vi "Instantiate.vi"(11 "error in":errorcluster) -> (4 "function manager":refnum<class "function manager.lvclass">, 15 "error out":errorcluster)   [LabVIEW 2016, in "function manager.lvclass"]
uses:
  function manager.lvclass
  functionsbase/functionbase.lvclass
  function manager.lvclass/function manager.ctl
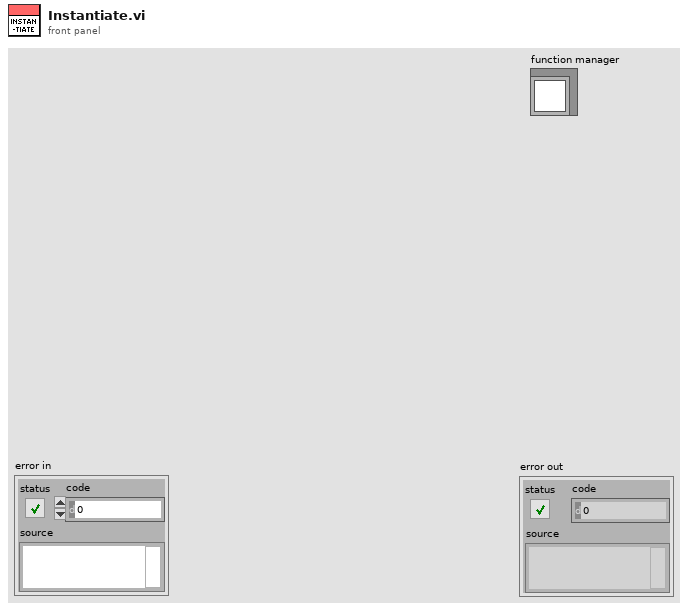
[diagram p1: front panel]
types:
  T1 = typedef "Scan Syntax Format.ctl" = cluster{"Syntax":string, "Variable#":i32, "Variables Name":string[]}
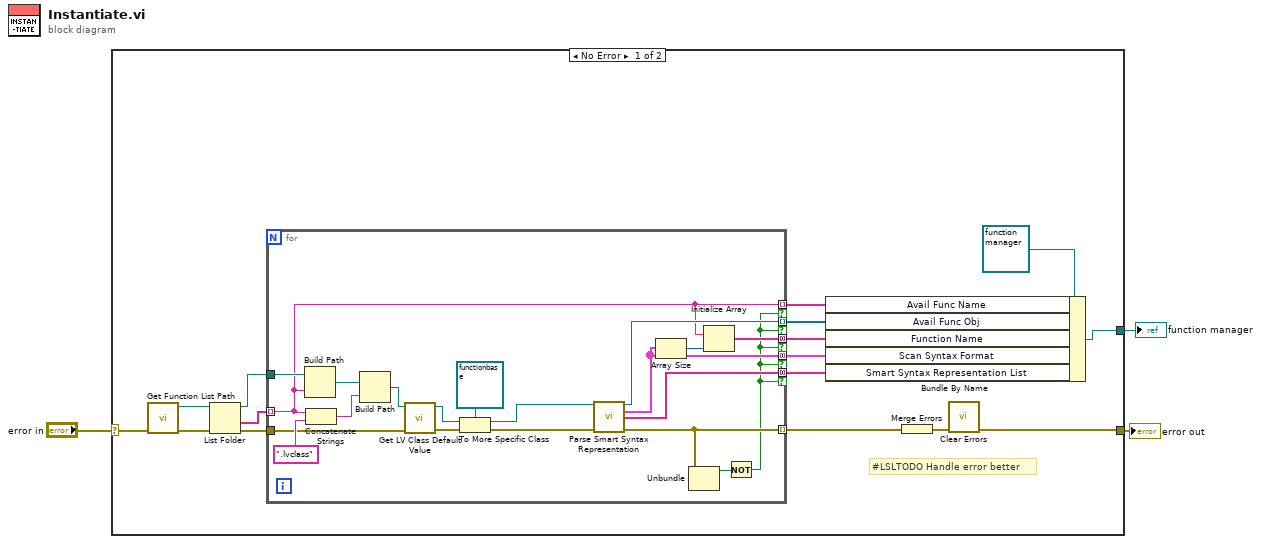
[diagram p0: block diagram]
diagram:
  n1 = case shown="No Error" "error in" {
    selector: "error in" -> [w19 w40]
    tunnel: [w11 w40] -> w2
    tunnel: [w7 _] -> w1
    frame No Error {
      # "#LSLTODO Handle error better"
      n2 = call "Get Function List Path.vi"("error in"=w19) -> ("error out"=w18:errorcluster, "Functions List Path"=w17:path)  [unwired: 9 in]
      n3 = List Folder(path=w17, error in=w18) -> (path out=w14:path, folder names=w15:string[], error out=w16:errorcluster)  [unwired: 2 in, 1 out]
      n4 = for {
        tunnel: w16 -> [w34]
        tunnel: w15 -> [w23] mode=indexing
        tunnel: w14 -> [w39]
        tunnel: [w28] -> w13 mode=indexing
        tunnel: [w26] -> w8 mode=indexing if=w20
        tunnel: [w23] -> w9 mode=indexing if=w20
        tunnel: [w25] -> w5 mode=concatenating if=w20
        tunnel: [w22] -> w6 mode=concatenating if=w20
        tunnel: [w21] -> w4 mode=concatenating if=w20
        n5 = Build Path(base path=w39, name or relative path=w23) -> (appended path=w38:path)
        n6 = Concatenate Strings(w23, ".lvclass" ("string")) -> (w36:string)
        n7 = Build Path(base path=w38, name or relative path=w36) -> (appended path=w35:path)
        n8 = call <vilib>:"Get LV Class Default Value.vi"("error in (no error)"=w34, "class path"=w35) -> ("error out"=w33:errorcluster, "object"=w32:refnum<class>)  [unwired: 8 in]
        n9 = To More Specific Class(target class=refnum<class "functionbase.lvclass"> refnum ("functionbase.lvclass"), reference=w32, error in=w33) -> (specific class reference=w27:refnum<class "functionbase.lvclass">, error out=w29:errorcluster)
        n10 = call-dynamic "Parse Smart Syntax Representation.vi"("functionbase in"=w27, "error in (no error)"=w29) -> ("functionbase out"=w26:refnum<class "functionbase.lvclass">, "Scan Syntax List"=w25:T1[], "Smart Syntax Representation List"=w21:string[], "error out"=w28:errorcluster)  [unwired: 10 in]
        n11 = Array Size(array=w25) -> (size(s)=w24:i32)
        n12 = Unbundle(w28) -> ("status"=w30:bool)  [unwired: 2 out]
        n13 = Initialize Array(w23, w24) -> (w22:string[])
        n14 = Not(x=w30) -> (.not. x?=w20:bool)
      }
      n15 = Bundle By Name(cluster=refnum<class "function manager.lvclass"> refnum ("function manager.lvlib:function manager.lvclass"), "Avail Func Name"=w9, "Avail Func Obj"=w8, "Function Name"=w6, "Scan Syntax Format"=w5, "Smart Syntax Representation List"=w4) -> (w7:refnum<class "function manager.lvclass">)
      n16 = Merge Errors(w13) -> (w12:errorcluster)
      n17 = call <vilib>:"Clear Errors.vi"("error in (no error)"=w12) -> ("error out"=w11:errorcluster)  [unwired: 5 in, 1 out]
    }
    frame Error {
    }
  }
  "error out" <- w2
  "function manager" <- w1
